vi "IntermediatePositions.vi"(1 "Dead Zone":dbl, 2 "Position Grids":T1=[{"x1"=0.0, "x2"=1.75, "resolution"=0.15}, {"x1"=1.75, "x2"=7.38, "resolution"=0.4}]) -> (0 "Positions":cluster{dbl, dbl}[](array[cluster]))   [LabVIEW 2015, in "Navigation2017.lvlib" / "SubVIs - Navigation2017.lvlib"]
uses:
  SubVIs - Navigation2017.lvlib
  IntermediatePositionGrids.ctl
  Navigation2017.lvlib
  Types - Navigation2017.lvlib
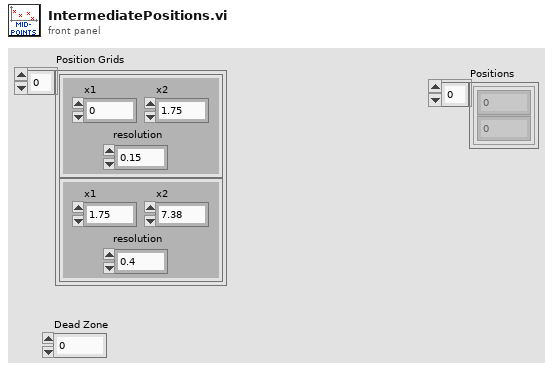
[diagram p1: front panel]
types:
  T1 = typedef "Navigation2017.lvlib/Types - Navigation2017.lvlib/IntermediatePositionGrids.ctl" = cluster{"x1":dbl, "x2":dbl, "resolution":dbl}[]
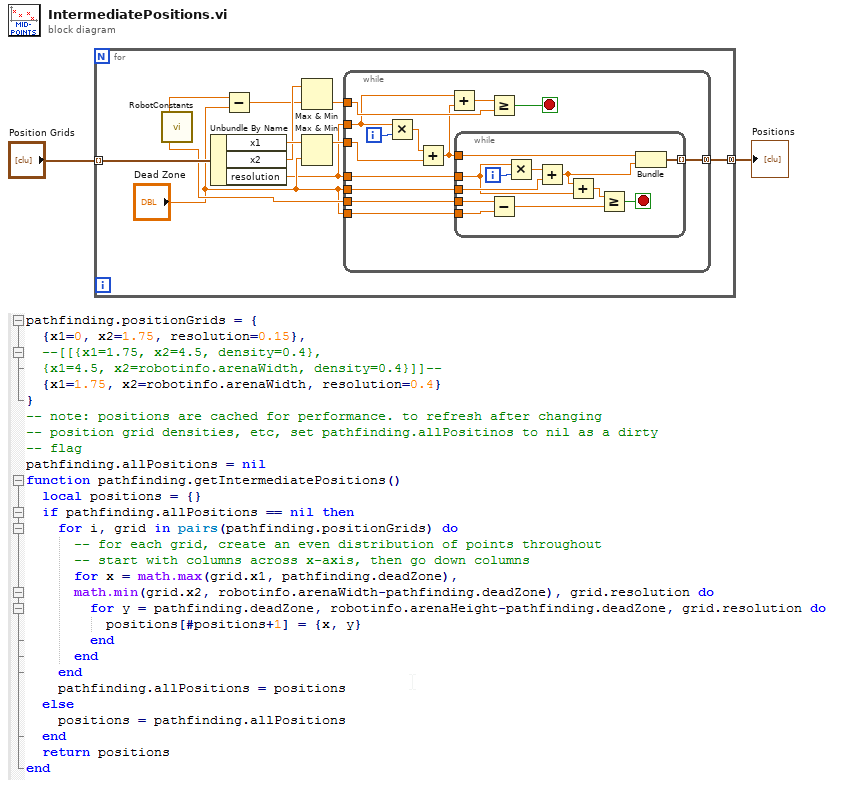
[diagram p0: block diagram]
diagram:
  n1 = for {
    tunnel: "Position Grids" -> [w13] mode=indexing
    tunnel: [w3] -> w1 mode=concatenating
    n2 = call "RobotConstants.vi"() -> ("Arena Width (m)"=w9:dbl, "Arena Height (m)"=w6:dbl)  [unwired: 3 out]
    n3 = Unbundle By Name(w13) -> ("x1"=w12:dbl, "x2"=w11:dbl, "resolution"=w4:dbl)
    n4 = Subtract(x=w9, y="Dead Zone") -> (x-y=w10:dbl)
    n5 = Max & Min(x=w11, y=w10) -> (min(x,y)=w7:dbl)  [unwired: 1 out]
    n6 = Max & Min(x=w12, y="Dead Zone") -> (max(x,y)=w8:dbl)  [unwired: 1 out]
    n7 = while {
      tunnel: w8 -> [w26]
      tunnel: w4 -> [w15]
      tunnel: w7 -> [w22]
      tunnel: "Dead Zone" -> [w21]
      tunnel: w6 -> [w20]
      tunnel: "Dead Zone" -> [w19]
      tunnel: w4 -> [w18]
      tunnel: [w17] -> w3 mode=concatenating
      i -> [w25]
      stop <- w23 stop-if-true
      n8 = Multiply(x=w15, y=w25) -> (x*y=w24:dbl)
      n9 = Add(x=w24, y=w26) -> (x+y=w14:dbl)
      n10 = Add(x=w15, y=w14) -> (x+y=w16:dbl)
      n11 = while {
        tunnel: w21 -> [w35]
        tunnel: w20 -> [w33]
        tunnel: w19 -> [w32]
        tunnel: w18 -> [w27]
        tunnel: w14 -> [w31]
        tunnel: [w30] -> w17 mode=indexing
        i -> [w36]
        stop <- w37 stop-if-true
        n12 = Subtract(x=w33, y=w32) -> (x-y=w34:dbl)
        n13 = Multiply(x=w27, y=w36) -> (x*y=w38:dbl)
        n14 = Add(x=w38, y=w35) -> (x+y=w28:dbl)
        n15 = Add(x=w28, y=w27) -> (x+y=w29:dbl)
        n16 = Greater Or Equal?(x=w29, y=w34) -> (x >= y?=w37:bool)
        n17 = Bundle(w31, w28) -> (w30:cluster{dbl, dbl})  [unwired: 1 in]
      }
      n18 = Greater Or Equal?(x=w16, y=w22) -> (x >= y?=w23:bool)
    }
  }
  "Positions" <- w1
